vi "Create Base Queue.vi"(9 "Queue":refnum<class "Queue.lvclass">, 10 "Self Queue Alias":string) -> (0 "error out":errorcluster)   [LabVIEW 2021, in "jettl.lvlib" / "Base Queue.lvlib"]
uses:
  Base Queue.lvlib
  Queue/Queue.lvclass
  Base Queue/Base Queue.lvclass
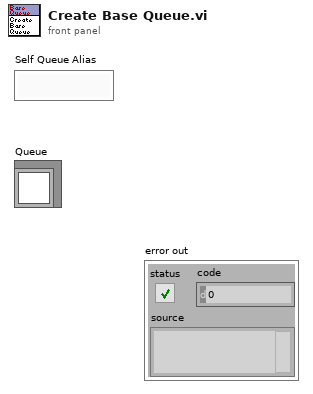
[diagram p1: front panel]
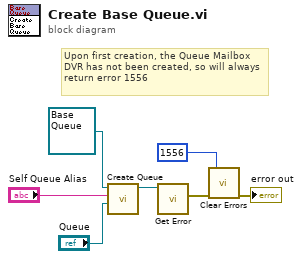
[diagram p0: block diagram]
diagram:
  # "Upon first creation, the Queue Mailbox DVR has not been created, so will always return error 1556"
  n1 = call-dynamic "Create Queue.vi"("Queue"="Queue", "Self Queue Alias"="Self Queue Alias", "Base Queue in"=refnum<class "Base Queue.lvclass"> refnum ("jettl Queue Actor.lvlib:jettl Queue Actor.lvclass")) -> ("Base Queue out"=w6:refnum<class "Base Queue.lvclass">)  [unwired: 8 in]
  n2 = call-dynamic "Get Error.vi"("Base Queue in"=w6) -> ("Error"=w2:errorcluster)  [unwired: 10 in]
  n3 = call <vilib>:"Clear Errors.vi"("error in (no error)"=w2, "specific error code to clear (0: all)"=1556) -> ("error out"=→"error out":errorcluster)  [unwired: 4 in, 1 out]
